vi "Autonomous.vi"() -> ()   [LabVIEW 2016]
doc: "This VI starts when autonomous period begins, and will automatically be terminated when it ends. You can carry out timed or sensor driven operations directly to I/O or to subsystems without needing to return to the caller."
uses:
  <vilib>/Rock Robotics/WPI/Solenoid/WPI_SolenoidValue.ctl
  <vilib>/Rock Robotics/Network Tables/NT Read String.vi
  <vilib>/Rock Robotics/Network Tables/NT Read Number.vi
  <vilib>/Rock Robotics/WPI/Solenoid/WPI_SolenoidSetEnum.vi
  Drive/Implementation/Drive Published Globals.vi
panel:
  in  "motor test time":dbl=1.0
  in  "Suckit":dbl=0.15 format="%#_13g"
  in  "Distance (ft) 2":dbl=3.0 format="%#_13g"
  in  "Distance (ft) 5":dbl=1.5
  in  "Distance (ft) 4":dbl=3.0
  in  "Distance (ft)":dbl=3.0 format="%#_13g"
  in  "Secs for flywheel spinup":dbl=0.3
  in  "Seconds to score":dbl=0.75
  in  "speed of backing up":dbl=0.3 format="%#_13g"
  in  "Seconds of backing up":dbl=2.0 format="%#_13g"
  in  "speed":dbl=-0.5 format="%#_13g"
  in  "Distance to go Forward":dbl=-11.658 format="%#_13g"
  in  "Score Goal Wait":dbl=0.5
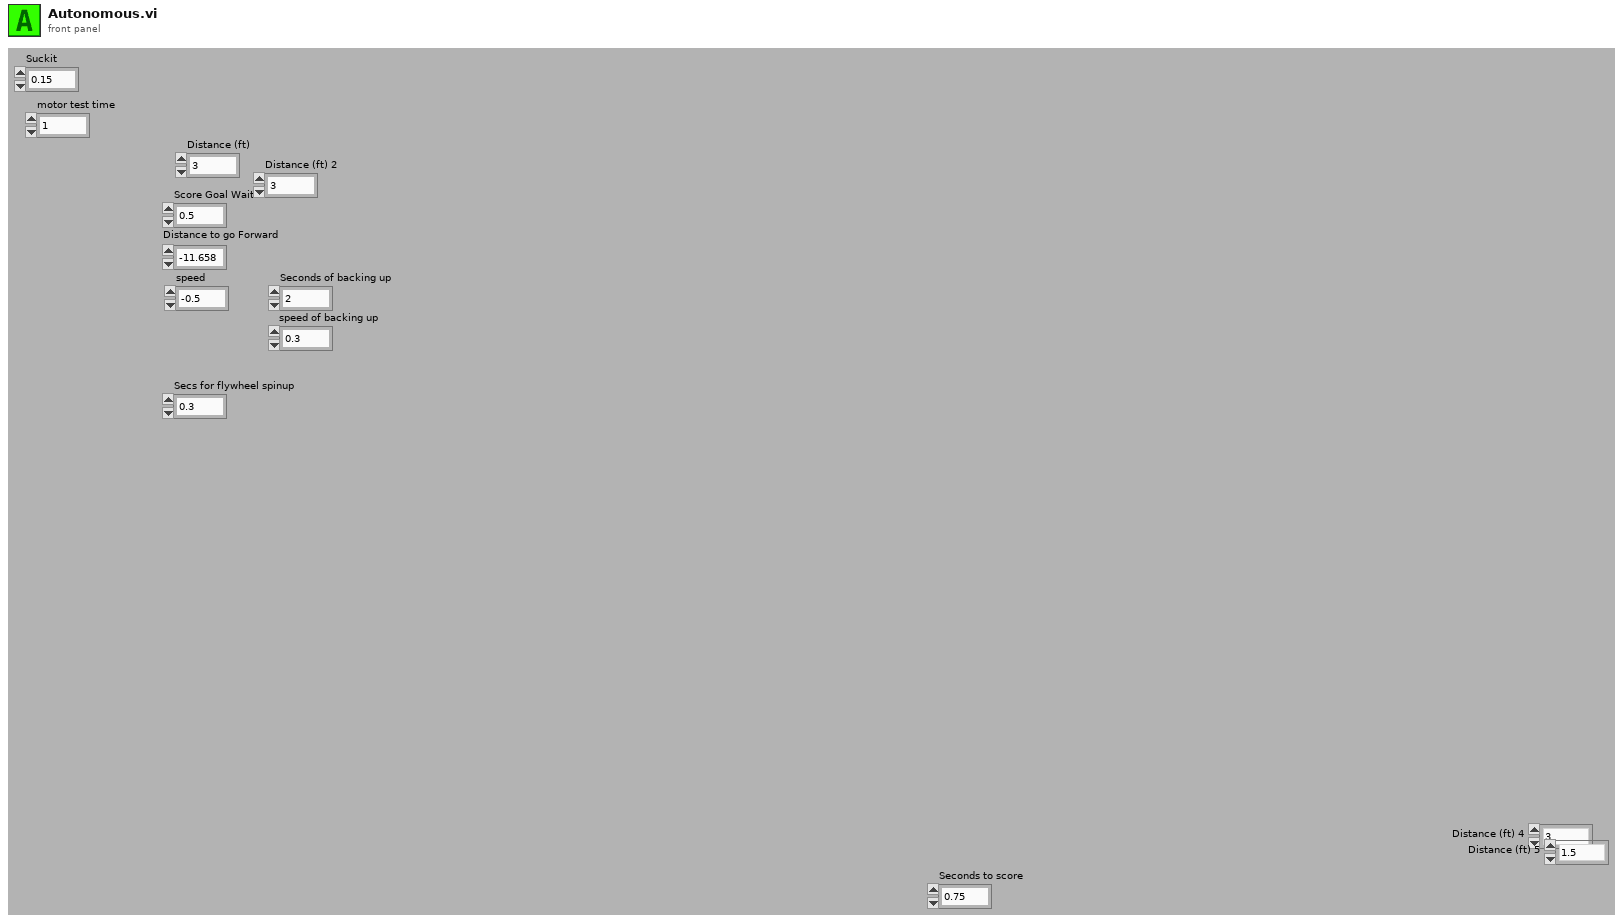
[diagram p1: front panel]
types:
  T1 = typedef "WPI_MotorControlDeviceRef.ctl" = cluster{"DeviceStatus":errorcluster, "Type":T2, "PWM":cluster{"PWM Channel":T3, "DeadBand":T4}, "CAN":cluster{"Device Number":u8, "SetOutput VI Ref":variant, "GetOutput VI Ref":variant, "Enable VI Ref":variant, "Disable VI Ref":variant, "Data":variant}, "Invert":bool}
  T2 = typedef "WPI_MotorControlType.ctl" = enum16{"PWM", "CAN"}
  T3 = typedef "FPGA_DIOPWMChannel.ctl" = enum8{"PWM 0", "PWM 1", "PWM 2", "PWM 3", "PWM 4", "PWM 5", "PWM 6", "PWM 7", "PWM 8", "PWM 9", "PWM MXP 0", "PWM MXP 1", "PWM MXP 2", "PWM MXP 3", "PWM MXP 4", "PWM MXP 5", "PWM MXP 6", "PWM MXP 7", "PWM MXP 8", "PWM MXP 9", "Invalid"}
  T4 = typedef "WPI_PWMDeadband.ctl" = cluster{"Name":string, "maxPositivePwm":i32, "minPositivePwm":i32, "centerPwm":i32, "maxNegativePwm":i32, "minNegativePwm":i32, "angularRange":u16}
  T5 = typedef "WPI_SolenoidDevRef.ctl" = cluster{"DevStatus":errorcluster, "Pneumatics Control Module":u8, "Forward Solenoid Channel":T6, "Reverse Solenoid Channel":T6}
  T6 = typedef "WPI_SolenoidChannel.ctl" = enum8{"Solenoid 0", "Solenoid 1", "Solenoid 2", "Solenoid 3", "Solenoid 4", "Solenoid 5", "Solenoid 6", "Solenoid 7", "Invalid"}
  T7 = typedef "WPI_SolenoidValue.ctl" = enum16{"Off", "On", "Forward", "Reverse"}
  T8 = typedef "Command Status Info.ctl" = cluster{"Name":string, "Status":T9, "notifier out":T10}
  T9 = typedef "Completion Status.ctl" = enum16{"Successful", "Aborted", "Incomplete"}
  T10 = typedef "Completion Notifier.ctl" = refnum<notifier>
  T11 = typedef "CTRE_PigeonIMU_DeviceRef.ctl" = cluster{"DeviceStatus":errorcluster, "Device Number":u8, "Type":T12, "Device ID":u32}
  T12 = typedef "CTRE_PigeonIMU_ConnectionType.ctl" = u32
  T13 = typedef "CTRE_PigeonIMU_GlobalStatus.ctl" = cluster{"PigeonState":T14, "FusedHeading":cluster{"Heading":dbl, "Valid?":bool, "Fusing?":bool}, "YPR":cluster{"Yaw":dbl, "Pitch":dbl, "Roll":dbl}, "Compass":cluster{"Heading":dbl, "Magnitude":dbl, "Absolute Heading":dbl}, "Accelerometer":cluster{"Biased":cluster{"X":i16, "Y":i16, "Z":i16, "Norm":i16}, "Angles":cluster{"XZ Tilt":dbl, "YZ Tilt":dbl, "XY Tilt":dbl}}, "Magnetometer":cluster{"Raw":cluster{"X":i16, "Y":i16, "Z":i16}, "Biased":cluster{"X":i16, "Y":i16, "Z":i16}}, "Gyro":cluster{"X":dbl, "Y":dbl, "Z":dbl, "Norm":dbl}, "6D Quaternian":cluster{"W":dbl, "X":dbl, "Y":dbl, "Z":dbl}, "Temp. (C)":dbl, "UpTime":u32, "StartupStatus":cluster{"ResetCount":i32, "ResetFlags":i32, "FirmwareVersion":i32, "HasReset?":bool}, "Calibration":cluster{"CurrentMode":T15, "LastCalError":i32, "CalBooting?":bool}, "CAN Error":errorcluster, "AccumGyro":cluster{"X":dbl, "Y":dbl, "Z":dbl}, "Usage Frame":u32}
  T14 = typedef "CTRE_PigeonIMU_PigeonState.ctl" = enum16{"NoComm", "Initializing", "Ready", "UserCalibration"}
  T15 = typedef "CTRE_PigeonIMU_CalibrationMode.ctl" = u16
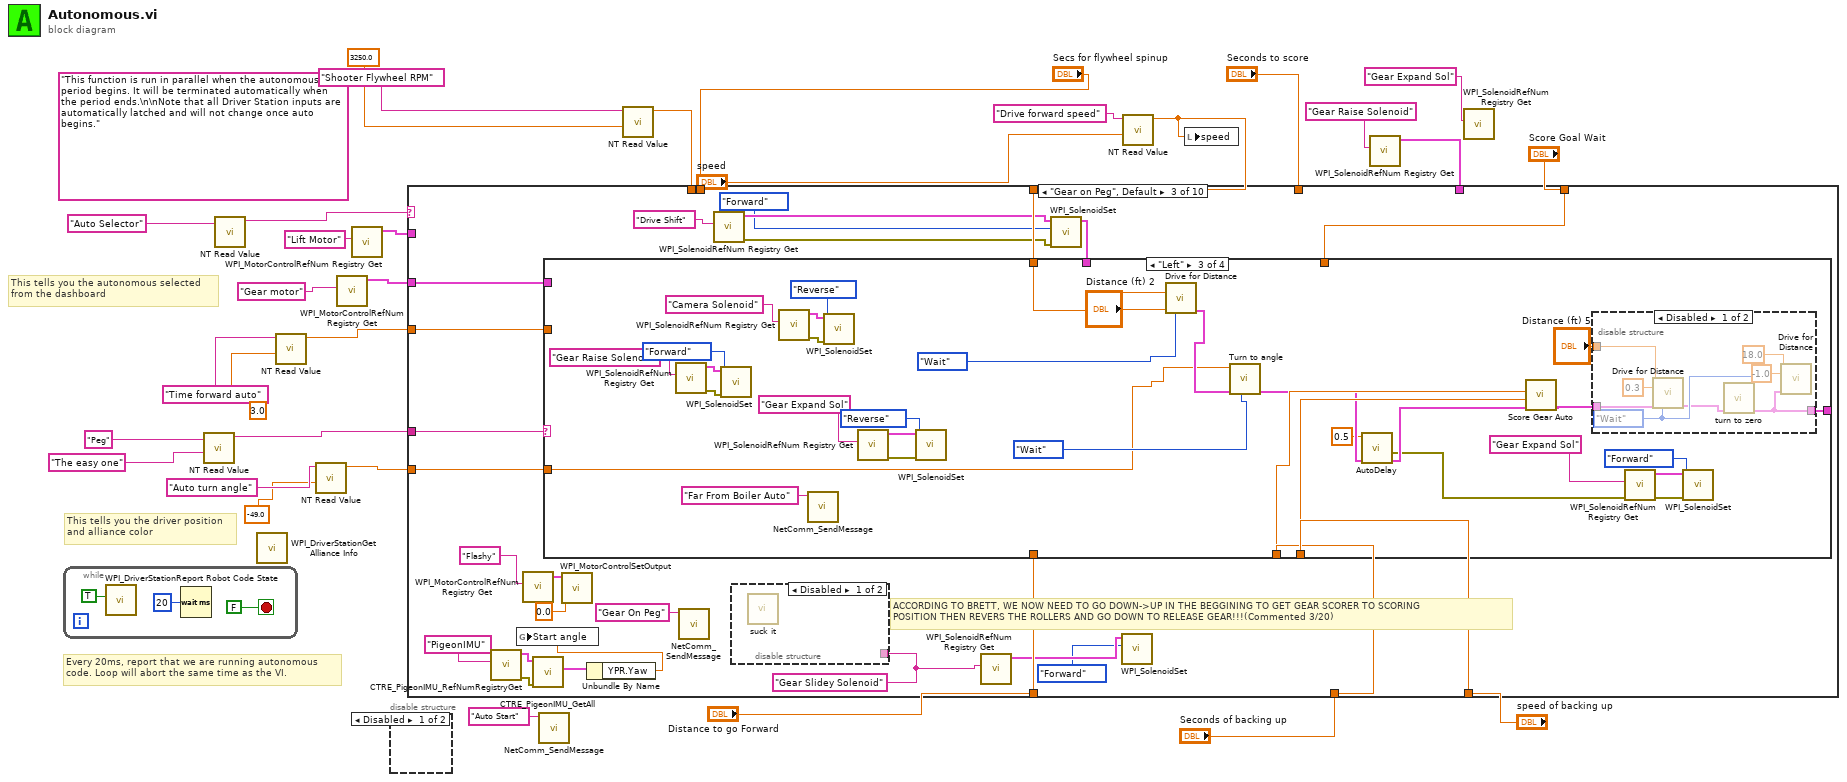
[diagram p0: block diagram]
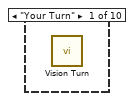
[diagram p3: hidden frame]
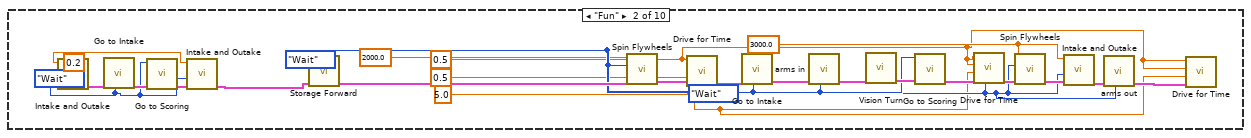
[diagram p4: hidden frame]
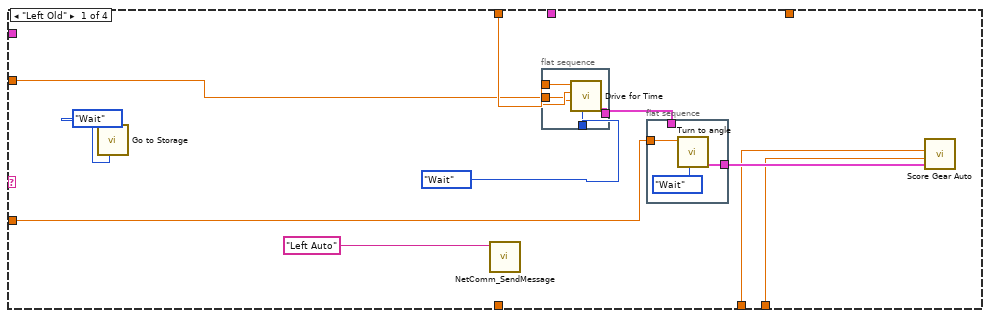
[diagram p6: hidden frame]
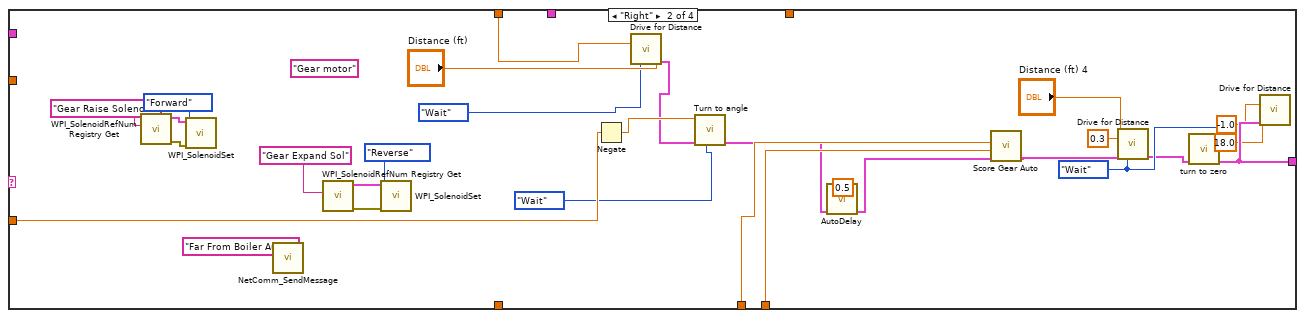
[diagram p7: hidden frame]
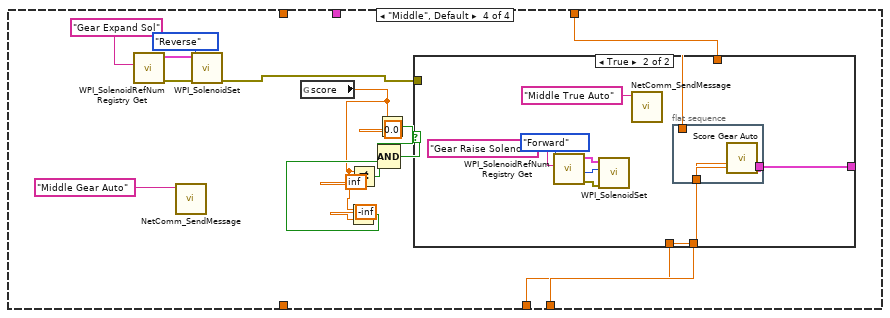
[diagram p9: hidden frame]
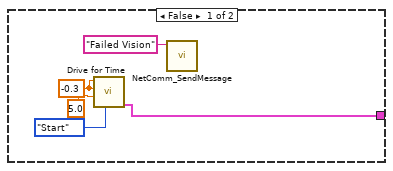
[diagram p10: hidden frame]
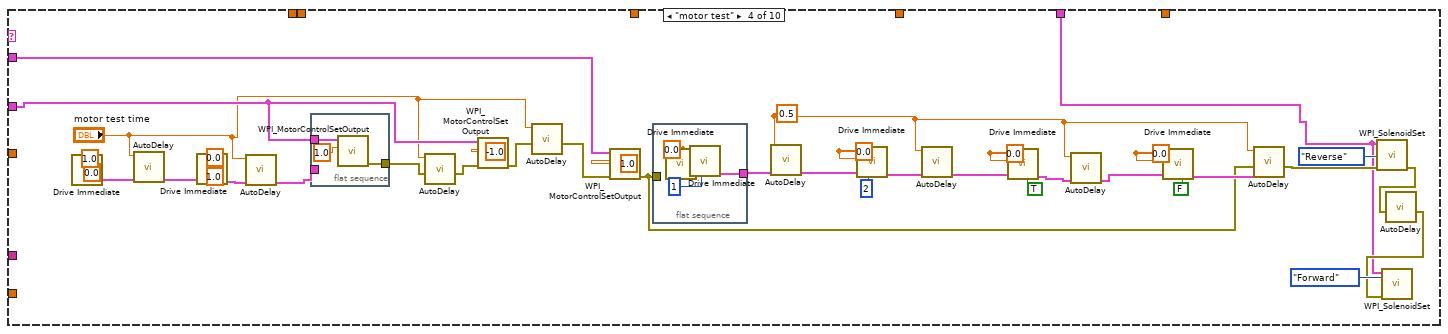
[diagram p11: hidden frame]
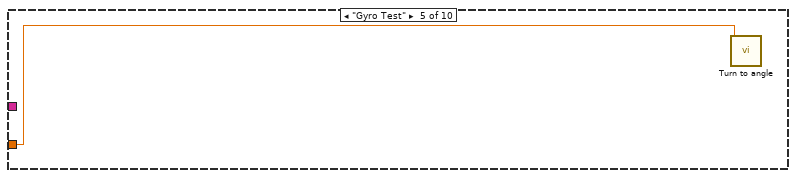
[diagram p12: hidden frame]
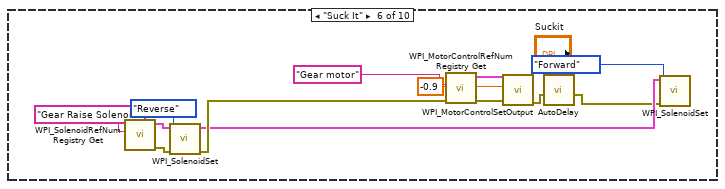
[diagram p13: hidden frame]
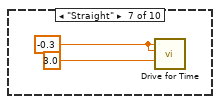
[diagram p14: hidden frame]
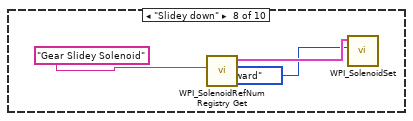
[diagram p15: hidden frame]
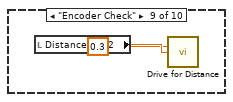
[diagram p16: hidden frame]
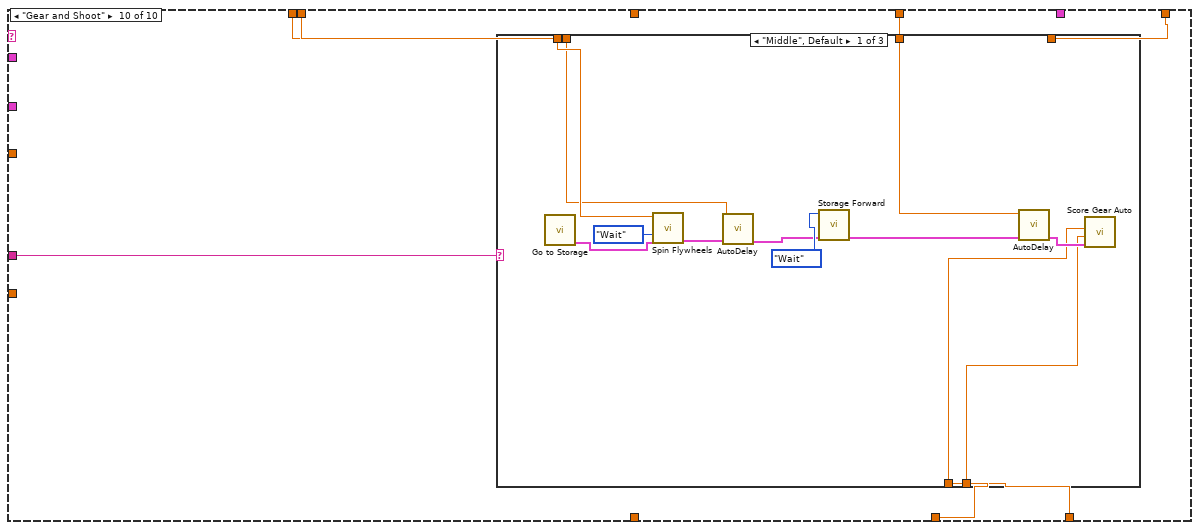
[diagram p17: hidden frame]
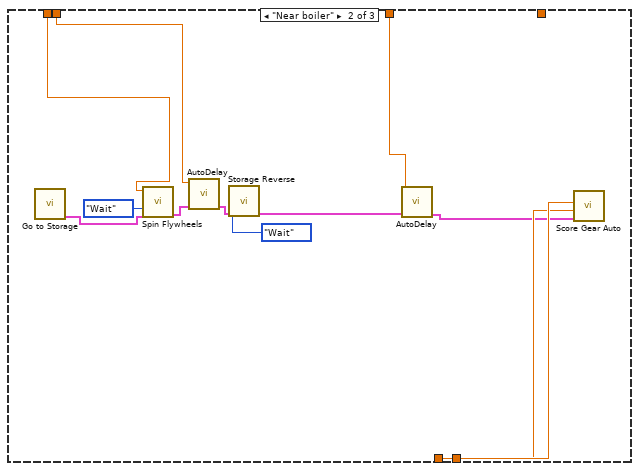
[diagram p18: hidden frame]
diagram:
  (unwired) "This function is run in parallel when the autonomous period begins. It will be terminated automatically when the period ends.\n\nNote that all Driver Station inputs are automatically latched and will not change once auto begins."
  # "This tells you the autonomous selected\nfrom the dashboard"
  # "Every 20ms, report that we are running autonomous\ncode. Loop will abort the same time as the VI."
  # "This tells you the driver position\nand alliance color"
  n1 = while {
    stop <- FALSE stop-if-true
    n2 = call <vilib>:"WPI_DriverStationReport Robot Code State.vi"("Autonomous"=TRUE) -> ()  [unwired: 10 in, 1 out]
    n3 = Wait (ms)(milliseconds to wait=u32 20) -> ()  [unwired: 1 out]
  }
  n4 = call-poly <vilib>:"NT Read Value.vi"("Default Value"="The easy one", "Name"="Peg") -> ("String"=w27:string)  [unwired: 8 in, 1 out]
  n5 = call-poly <vilib>:"NT Read Value.vi"("Name"="Auto Selector") -> ("String"=w30:string)  [unwired: 9 in, 1 out]
  n6 = call <vilib>:"WPI_DriverStationGet Alliance Info.vi"() -> ()  [unwired: 12 out]
  n7 = call-poly <vilib>:"NT Read Value.vi"("Default Value"=3.0, "Name"="Time forward auto") -> ("Numeric"=w15:dbl)  [unwired: 8 in, 1 out]
  n8 = call-poly <vilib>:"NT Read Value.vi"("Default Value"=-49.0, "Name"="Auto turn angle") -> ("Numeric"=w12:dbl)  [unwired: 8 in, 1 out]
  n9 = call <vilib>:"WPI_MotorControlRefNum Registry Get.vi"("refnum name"="Gear motor") -> ("MotorControlDevRef"=w7:T1)  [unwired: 9 in, 1 out]
  n10 = call <vilib>:"WPI_MotorControlRefNum Registry Get.vi"("refnum name"="Lift Motor") -> ("MotorControlDevRef"=w4:T1)  [unwired: 9 in, 1 out]
  n11 = disable-structure shown="Disabled" {
    frame Disabled {
    }
    frame Enabled {
    }
  }
  n12 = call <vilib>:"NetComm_SendMessage.vi"("Message"="Auto Start") -> ()  [unwired: 11 in]
  n13 = call-poly <vilib>:"NT Read Value.vi"("Default Value"=3250.0, "Name"="Shooter Flywheel RPM") -> ("Numeric"=w18:dbl)  [unwired: 8 in, 1 out]
  n14 = call-poly <vilib>:"NT Read Value.vi"("Default Value"="speed", "Name"="Drive forward speed") -> ("Numeric"=w9:dbl)  [unwired: 8 in, 1 out]
  n15 = local write "speed"(w9) -> ()
  n16 = call <vilib>:"WPI_SolenoidRefNum Registry Get.vi"("refnum name"="Gear Raise Solenoid") -> ("SolenoidDevRef"=w1:T5)  [unwired: 9 in, 1 out]
  n17 = case shown="\"Gear on Peg\", Default" w30 {
    tunnel: w27 -> [_ _ w84 _ _ _ _ _ _ w277]
    tunnel: w9 -> [_ _ w83 _ _ _ _ _ _ _]
    tunnel: "Distance to go Forward" -> [_ _ w82 _ _ _ _ _ _ _]
    tunnel: "speed of backing up" -> [_ _ w81 _ _ _ _ _ _ w275]
    tunnel: "Seconds of backing up" -> [_ _ w80 _ _ _ _ _ _ w276]
    tunnel: "Score Goal Wait" -> [_ _ w79 _ _ _ _ _ _ w274]
    tunnel: "Seconds to score" -> [_ _ _ _ _ _ _ _ _ w273]
    tunnel: "Secs for flywheel spinup" -> [_ _ _ _ _ _ _ _ _ w272]
    tunnel: w18 -> [_ _ _ _ _ _ _ _ _ w271]
    tunnel: w15 -> [_ _ w78 _ _ _ _ _ _ _]
    tunnel: w12 -> [_ _ w77 _ w249 _ _ _ _ _]
    tunnel: w7 -> [_ _ w71 w231 _ _ _ _ _ _]
    tunnel: w4 -> [_ _ _ w228 _ _ _ _ _ _]
    tunnel: w1 -> [_ _ _ w205 _ _ _ _ _ _]
    frame "Your Turn" {
      n18 = call "Vision Turn.vi"() -> ()  [unwired: 11 in, 1 out]
    }
    frame "Fun" {
      w36 = enum16{"Start", "Wait"}."Wait" ("Synchronication")
      w35 = 0.2 ("Speed")
      w47 = 3000.0 ("Speed RPM")
      w44 = enum16{"Start", "Wait"}."Wait" ("Synchronization")
      w41 = 5.0 ("Seconds")
      w42 = 0.5 ("Left Speed")
      w52 = enum16{"Start", "Wait"}."Wait" ("Synchronication")
      n19 = call "Intake and Outake.vi"("Synchronication"=w36, "Speed"=w35) -> ("Command Info Out"=w40:T8)  [unwired: 9 in]
      n20 = call "Go to Intake.vi"("Synchronication"=w36, "Command Info In"=w40) -> ("Command Info Out"=w38:T8)  [unwired: 9 in]
      n21 = call "Go to Scoring.vi"("Command Info In"=w38, "Synchronication"=w36) -> ("Command Info Out"=w37:T8)  [unwired: 9 in]
      n22 = call "Intake and Outake.vi"("Command Info In"=w37, "Synchronication"=w36, "Speed"=w35) -> ("Command Info Out"=w39:T8)  [unwired: 8 in]
      n23 = call "Storage Forward.vi"("Command Info In"=w39, "Synchronication"=w52) -> ("Command Info Out"=w58:T8)  [unwired: 9 in]
      n24 = call "Spin Flywheels.vi"("Command Info In"=w58, "Synchronication"=w52, "Speed RPM"=2000.0) -> ("Command Info Out"=w57:T8)  [unwired: 8 in]
      n25 = call "Drive for Time.vi"("Synchronization"=w52, "Command Info In"=w57, "Seconds"=w41, "Right Speed"=0.5, "Left Speed"=w42) -> ("Command Info Out"=w56:T8)  [unwired: 4 in, 2 out]
      n26 = call "Go to Intake.vi"("Synchronication"=w52, "Command Info In"=w56) -> ("Command Info Out"=w55:T8)  [unwired: 9 in]
      n27 = call "arms in.vi"("Synchronication"=w52, "Command Info In"=w55) -> ("Command Info Out"=w54:T8)  [unwired: 9 in]
      n28 = call "Vision Turn.vi"("Command Info In"=w54) -> ("Command Info Out"=w53:T8)  [unwired: 10 in]
      n29 = call "Go to Scoring.vi"("Command Info In"=w53, "Synchronication"=w52) -> ("Command Info Out"=w50:T8)  [unwired: 9 in]
      n30 = call "Drive for Time.vi"("Synchronization"=w44, "Command Info In"=w50, "Seconds"=w41, "Right Speed"=w42, "Left Speed"=w42) -> ("Command Info Out"=w48:T8)  [unwired: 4 in, 2 out]
      n31 = call "Spin Flywheels.vi"("Command Info In"=w48, "Synchronication"=w44, "Speed RPM"=w47) -> ("Command Info Out"=w46:T8)  [unwired: 8 in]
      n32 = call "Intake and Outake.vi"("Command Info In"=w46, "Synchronication"=w44, "Speed"=w47) -> ("Command Info Out"=w45:T8)  [unwired: 8 in]
      n33 = call "arms out.vi"("Synchronication"=w44, "Command Info In"=w45) -> ("Command Info Out"=w43:T8)  [unwired: 9 in]
      n34 = call "Drive for Time.vi"("Command Info In"=w43, "Seconds"=w41, "Right Speed"=w42, "Left Speed"=w42) -> ()  [unwired: 5 in, 3 out]
    }
    frame "Gear on Peg", Default {
      w62 = "Gear Slidey Solenoid" ("refnum name")
      # "ACCORDING TO BRETT, WE NOW NEED TO GO DOWN->UP IN THE BEGGINING TO GET GEAR SCORER TO SCORING \nPOSITION THEN REVERS THE ROLLERS AND GO DOWN TO RELEASE GEAR!!!(Commented 3/20)"
      n35 = call <vilib>:"CTRE_PigeonIMU_RefNumRegistryGet.vi"("refnum name"="PigeonIMU") -> ("error out"=w68:errorcluster, "PigeonIMUDevRef"=w67:T11)  [unwired: 9 in]
      n36 = call <vilib>:"WPI_MotorControlRefNum Registry Get.vi"("refnum name"="Flashy") -> ("MotorControlDevRef"=w60:T1)  [unwired: 9 in, 1 out]
      n37 = call <vilib>:"CTRE_PigeonIMU_GetAll.vi"("error in (no error)"=w68, "PigeonIMUDevRef"=w67) -> ("Get All"=w66:T13)  [unwired: 7 in, 2 out]
      n38 = call <vilib>:"WPI_MotorControlSetOutput.vi"("Output"=0.0, "MotorControlDevRef"=w60) -> ()  [unwired: 7 in, 3 out]
      n39 = Unbundle By Name(w66) -> ("YPR.Yaw"=w65:dbl)
      n40 = global write "Drive Published Globals.vi" "Start angle"(w65) -> ()
      n41 = call <vilib>:"NetComm_SendMessage.vi"("Message"="Gear On Peg") -> ()  [unwired: 11 in]
      n42 = call <vilib>:"WPI_SolenoidRefNum Registry Get.vi"("refnum name"="Drive Shift") -> ("error out"=w74:errorcluster, "SolenoidDevRef"=w75:T5)  [unwired: 9 in]
      n43 = disable-structure shown="Disabled" {
        disable-tunnel: w62 -> [_ _]
        frame Disabled {
          n44 = call "suck it.vi"() -> ()  [unwired: 12 in]
        }
        frame Enabled {
        }
      }
      n45 = call <vilib>:"WPI_SolenoidRefNum Registry Get.vi"("refnum name"=w62) -> ("SolenoidDevRef"=w64:T5)  [unwired: 9 in, 1 out]
      n46 = call-poly <vilib>:"WPI_SolenoidSet.vi"("error in (no error)"=w74, "Value"=WPI_SolenoidValue."Forward", "SolenoidDevRef"=w75) -> ("SolenoidDevRef"=w72:T5)  [unwired: 7 in, 1 out]
      n47 = case shown="\"Left\"" w84 {
        tunnel: w83 -> [w90 w113 w147 _]
        tunnel: w82 -> [_ _ _ _]
        tunnel: w81 -> [w93 w130 w162 w187]
        tunnel: w80 -> [w92 w129 w161 w186]
        tunnel: w79 -> [_ _ _ w185]
        tunnel: w78 -> [w89 _ _ _]
        tunnel: w77 -> [w91 w127 w140 _]
        tunnel: w72 -> [_ _ _ _]
        tunnel: w71 -> [_ _ _ _]
        tunnel: [_ w104 w141 _] -> _
        frame "Left Old" {
          n48 = call "Go to Storage.vi"("Synchronication"=enum16{"Start", "Wait"}."Wait") -> ()  [unwired: 10 in, 1 out]
          n49 = call <vilib>:"NetComm_SendMessage.vi"("Message"="Left Auto") -> ()  [unwired: 11 in]
          n50 = flat-sequence {
            tunnel: w90 -> [w101]
            tunnel: w89 -> [w100]
            tunnel: enum16{"Start", "Wait"}."Wait" ("Synchronication") -> [w99]
            tunnel: [w98] -> w87
            frame #0 {
              n51 = call "Drive for Time.vi"("Synchronization"=w99, "Seconds"=w100, "Right Speed"=w101, "Left Speed"=w101) -> ("Command Info Out"=w98:T8)  [unwired: 5 in, 2 out]
            }
          }
          n52 = flat-sequence {
            tunnel: [w97] -> w94
            tunnel: w91 -> [w95]
            tunnel: w87 -> [_]
            frame #0 {
              n53 = call "Turn to angle.vi"("Synchronication"=enum16{"Start", "Wait"}."Wait", "Angle"=w95) -> ("Command Info Out"=w97:T8)  [unwired: 9 in]
            }
          }
          n54 = call "Score Gear Auto.vi"("Command Info in"=w94, "speed of backing up"=w93, "Seconds of backing up"=w92) -> ()  [unwired: 8 in, 1 out]
        }
        frame "Right" {
          (unwired) "Gear motor" ("refnum name")
          w107 = enum16{"Start", "Wait"}."Wait" ("Synchronication")
          n55 = call <vilib>:"WPI_SolenoidRefNum Registry Get.vi"("refnum name"="Gear Raise Solenoid") -> ("error out"=w122:errorcluster, "SolenoidDevRef"=w123:T5)  [unwired: 9 in]
          n56 = call-poly <vilib>:"WPI_SolenoidSet.vi"("error in (no error)"=w122, "Value"=WPI_SolenoidValue."Forward", "SolenoidDevRef"=w123) -> ()  [unwired: 7 in, 2 out]
          n57 = call <vilib>:"NetComm_SendMessage.vi"("Message"="Far From Boiler Auto") -> ()  [unwired: 11 in]
          n58 = call <vilib>:"WPI_SolenoidRefNum Registry Get.vi"("refnum name"="Gear Expand Sol") -> ("error out"=w119:errorcluster, "SolenoidDevRef"=w118:T5)  [unwired: 9 in]
          n59 = call-poly <vilib>:"WPI_SolenoidSet.vi"("error in (no error)"=w119, "Value"=WPI_SolenoidValue."Reverse", "SolenoidDevRef"=w118) -> ()  [unwired: 7 in, 2 out]
          n60 = Negate(x=w127) -> (-x=w128:dbl)
          n61 = call "Drive for Distance.vi"("speed"=w113, "Distance (ft)"="Distance (ft)", "Synchronication"=enum16{"Start", "Wait"}."Wait") -> ("Command Info Out"=w111:T8)  [unwired: 12 in]
          n62 = call "Turn to angle.vi"("Synchronication"=enum16{"Start", "Wait"}."Wait", "Command Info In"=w111, "Angle"=w128) -> ("Command Info Out"=w116:T8)  [unwired: 8 in]
          n63 = call "AutoDelay.vi"("Command Info In"=w116, "Seconds to wait"=0.5) -> ("Command Info Out"=w115:T8)  [unwired: 8 in, 1 out]
          n64 = call "Score Gear Auto.vi"("Command Info in"=w115, "speed of backing up"=w130, "Seconds of backing up"=w129) -> ("Command Info Out"=w105:T8)  [unwired: 8 in]
          n65 = call "Drive for Distance.vi"("speed"=0.3, "Distance (ft)"="Distance (ft) 4", "Command Info In"=w105, "Synchronication"=w107) -> ("Command Info Out"=w106:T8)  [unwired: 11 in]
          n66 = call "turn to zero.vi"("Synchronication"=w107, "Command Info In"=w106) -> ("Command Info Out"=w104:T8)  [unwired: 9 in]
          n67 = call "Drive for Distance.vi"("speed"=-1.0, "Distance (ft)"=18.0, "Command Info In"=w104) -> ()  [unwired: 12 in, 1 out]
        }
        frame "Left" {
          n68 = call <vilib>:"WPI_SolenoidRefNum Registry Get.vi"("refnum name"="Gear Raise Solenoid") -> ("error out"=w156:errorcluster, "SolenoidDevRef"=w157:T5)  [unwired: 9 in]
          n69 = call-poly <vilib>:"WPI_SolenoidSet.vi"("error in (no error)"=w156, "Value"=WPI_SolenoidValue."Forward", "SolenoidDevRef"=w157) -> ()  [unwired: 7 in, 2 out]
          n70 = call <vilib>:"WPI_SolenoidRefNum Registry Get.vi"("refnum name"="Camera Solenoid") -> ("error out"=w138:errorcluster, "SolenoidDevRef"=w137:T5)  [unwired: 9 in]
          n71 = call <vilib>:"NetComm_SendMessage.vi"("Message"="Far From Boiler Auto") -> ()  [unwired: 11 in]
          n72 = call-poly <vilib>:"WPI_SolenoidSet.vi"("error in (no error)"=w138, "Value"=WPI_SolenoidValue."Reverse", "SolenoidDevRef"=w137) -> ()  [unwired: 7 in, 2 out]
          n73 = call <vilib>:"WPI_SolenoidRefNum Registry Get.vi"("refnum name"="Gear Expand Sol") -> ("error out"=w153:errorcluster, "SolenoidDevRef"=w152:T5)  [unwired: 9 in]
          n74 = call-poly <vilib>:"WPI_SolenoidSet.vi"("error in (no error)"=w153, "Value"=WPI_SolenoidValue."Reverse", "SolenoidDevRef"=w152) -> ()  [unwired: 7 in, 2 out]
          n75 = call "Drive for Distance.vi"("speed"=w147, "Distance (ft)"="Distance (ft) 2", "Synchronication"=enum16{"Start", "Wait"}."Wait") -> ("Command Info Out"=w145:T8)  [unwired: 12 in]
          n76 = call "Turn to angle.vi"("Synchronication"=enum16{"Start", "Wait"}."Wait", "Command Info In"=w145, "Angle"=w140) -> ("Command Info Out"=w150:T8)  [unwired: 8 in]
          n77 = call "AutoDelay.vi"("Command Info In"=w150, "Seconds to wait"=0.5) -> ("Command Info Out"=w149:T8, "error out (no error)"=w131:errorcluster)  [unwired: 8 in]
          n78 = call "Score Gear Auto.vi"("Command Info in"=w149, "speed of backing up"=w162, "Seconds of backing up"=w161) -> ("Command Info Out"=w142:T8)  [unwired: 8 in]
          n79 = disable-structure shown="Disabled" {
            disable-tunnel: "Distance (ft) 5" -> [w170 _]
            disable-tunnel: w142 -> [w166 _]
            disable-tunnel: [w165 _] -> w141
            frame Disabled {
              w168 = enum16{"Start", "Wait"}."Wait" ("Synchronication")
              n80 = call "Drive for Distance.vi"("speed"=0.3, "Distance (ft)"=w170, "Command Info In"=w166, "Synchronication"=w168) -> ("Command Info Out"=w167:T8)  [unwired: 11 in]
              n81 = call "turn to zero.vi"("Synchronication"=w168, "Command Info In"=w167) -> ("Command Info Out"=w165:T8)  [unwired: 9 in]
              n82 = call "Drive for Distance.vi"("speed"=-1.0, "Distance (ft)"=18.0, "Command Info In"=w165) -> ()  [unwired: 12 in, 1 out]
            }
            frame Enabled {
            }
          }
          n83 = call <vilib>:"WPI_SolenoidRefNum Registry Get.vi"("error in (no error)"=w131, "refnum name"="Gear Expand Sol") -> ("error out"=w133:errorcluster, "SolenoidDevRef"=w134:T5)  [unwired: 8 in]
          n84 = call-poly <vilib>:"WPI_SolenoidSet.vi"("error in (no error)"=w133, "Value"=WPI_SolenoidValue."Forward", "SolenoidDevRef"=w134) -> ()  [unwired: 7 in, 2 out]
        }
        frame "Middle", Default {
          n85 = call <vilib>:"WPI_SolenoidRefNum Registry Get.vi"("refnum name"="Gear Expand Sol") -> ("error out"=w174:errorcluster, "SolenoidDevRef"=w173:T5)  [unwired: 9 in]
          n86 = call <vilib>:"NetComm_SendMessage.vi"("Message"="Middle Gear Auto") -> ()  [unwired: 11 in]
          n87 = call-poly <vilib>:"WPI_SolenoidSet.vi"("error in (no error)"=w174, "Value"=WPI_SolenoidValue."Reverse", "SolenoidDevRef"=w173) -> ("error out"=w171:errorcluster)  [unwired: 7 in, 1 out]
          n88 = global read "Drive Published Globals.vi" "score"() -> (w178:dbl)
          n89 = Not Equal?(x=w178, y=-inf) -> (x != y?=w180:bool)
          n90 = Not Equal?(x=w178, y=inf) -> (x != y?=w179:bool)
          n91 = Not Equal?(x=w178, y=0.0) -> (x != y?=w182:bool)
          n92 = Compound Arithmetic op=AND(w182, w180, w179) -> (w183:bool)
          n93 = case shown="True" w183 {
            tunnel: w187 -> [_ w201]
            tunnel: w186 -> [_ w200]
            tunnel: w185 -> [_ w199]
            tunnel: [w189 w198] -> _
            tunnel: w171 -> [_ _]
            frame False {
              w192 = -0.3 ("Right Speed")
              n94 = call "Drive for Time.vi"("Synchronization"=enum16{"Start", "Wait"}."Start", "Seconds"=5.0, "Right Speed"=w192, "Left Speed"=w192) -> ("Command Info Out"=w189:T8)  [unwired: 5 in, 2 out]
              n95 = call <vilib>:"NetComm_SendMessage.vi"("Message"="Failed Vision") -> ()  [unwired: 11 in]
            }
            frame True {
              n96 = call <vilib>:"WPI_SolenoidRefNum Registry Get.vi"("refnum name"="Gear Raise Solenoid") -> ("error out"=w194:errorcluster, "SolenoidDevRef"=w195:T5)  [unwired: 9 in]
              n97 = call-poly <vilib>:"WPI_SolenoidSet.vi"("error in (no error)"=w194, "Value"=WPI_SolenoidValue."Forward", "SolenoidDevRef"=w195) -> ()  [unwired: 7 in, 2 out]
              n98 = call <vilib>:"NetComm_SendMessage.vi"("Message"="Middle True Auto") -> ()  [unwired: 11 in]
              n99 = flat-sequence {
                tunnel: w201 -> [w204]
                tunnel: w200 -> [w203]
                tunnel: w199 -> [_]
                tunnel: [w202] -> w198
                frame #0 {
                  n100 = call "Score Gear Auto.vi"("speed of backing up"=w204, "Seconds of backing up"=w203) -> ("Command Info Out"=w202:T8)  [unwired: 9 in]
                }
              }
            }
          }
        }
      }
      n101 = call-poly <vilib>:"WPI_SolenoidSet.vi"("Value"=WPI_SolenoidValue."Forward", "SolenoidDevRef"=w64) -> ()  [unwired: 8 in, 2 out]
    }
    frame "motor test" {
      w216 = 0.0 ("Left Setpoint")
      w220 = 0.0 ("Left Setpoint")
      w212 = 0.5 ("Seconds to wait")
      w224 = 0.0 ("Left Setpoint")
      n102 = call "Drive Immediate.vi"("Right Setpoint"=0.0, "Left Setpoint"=1.0) -> ("Command Info Out"=w241:T8)  [unwired: 9 in]
      n103 = call "AutoDelay.vi"("Command Info In"=w241, "Seconds to wait"="motor test time") -> ("Command Info Out"=w239:T8)  [unwired: 8 in, 1 out]
      n104 = call "Drive Immediate.vi"("Command Info In"=w239, "Right Setpoint"=1.0, "Left Setpoint"=0.0) -> ("Command Info Out"=w236:T8)  [unwired: 8 in]
      n105 = call "AutoDelay.vi"("Command Info In"=w236, "Seconds to wait"="motor test time") -> ("Command Info Out"=w235:T8)  [unwired: 8 in, 1 out]
      n106 = flat-sequence {
        tunnel: w231 -> [w248]
        tunnel: w235 -> [_]
        tunnel: [w247] -> w234
        frame #0 {
          n107 = call <vilib>:"WPI_MotorControlSetOutput.vi"("Output"=1.0, "MotorControlDevRef"=w248) -> ("error out"=w247:errorcluster)  [unwired: 7 in, 2 out]
        }
      }
      n108 = call "AutoDelay.vi"("error in (no error)"=w234, "Seconds to wait"="motor test time") -> ("error out (no error)"=w233:errorcluster)  [unwired: 8 in, 1 out]
      n109 = call <vilib>:"WPI_MotorControlSetOutput.vi"("error in (no error)"=w233, "Output"=-1.0, "MotorControlDevRef"=w231) -> ("error out"=w227:errorcluster)  [unwired: 6 in, 2 out]
      n110 = call "AutoDelay.vi"("error in (no error)"=w227, "Seconds to wait"="motor test time") -> ("error out (no error)"=w229:errorcluster)  [unwired: 8 in, 1 out]
      n111 = call <vilib>:"WPI_MotorControlSetOutput.vi"("error in (no error)"=w229, "Output"=1.0, "MotorControlDevRef"=w228) -> ("error out"=w210:errorcluster)  [unwired: 6 in, 2 out]
      n112 = flat-sequence {
        tunnel: w210 -> [_]
        tunnel: [w243] -> w223
        frame #0 {
          w245 = 0.0 ("Left Setpoint")
          n113 = call "Drive Immediate.vi"("Shift"=1, "Right Setpoint"=w245, "Left Setpoint"=w245) -> ("Command Info Out"=w243:T8)  [unwired: 8 in]
        }
      }
      n114 = call "Drive Immediate.vi"() -> ()  [unwired: 11 in, 1 out]
      n115 = call "AutoDelay.vi"("Command Info In"=w223, "Seconds to wait"=w212) -> ("Command Info Out"=w222:T8)  [unwired: 8 in, 1 out]
      n116 = call "Drive Immediate.vi"("Shift"=2, "Command Info In"=w222, "Right Setpoint"=w224, "Left Setpoint"=w224) -> ("Command Info Out"=w219:T8)  [unwired: 7 in]
      n117 = call "AutoDelay.vi"("Command Info In"=w219, "Seconds to wait"=w212) -> ("Command Info Out"=w221:T8)  [unwired: 8 in, 1 out]
      n118 = call "Drive Immediate.vi"("Brake"=TRUE, "Command Info In"=w221, "Right Setpoint"=w220, "Left Setpoint"=w220) -> ("Command Info Out"=w215:T8)  [unwired: 7 in]
      n119 = call "AutoDelay.vi"("Command Info In"=w215, "Seconds to wait"=w212) -> ("Command Info Out"=w214:T8)  [unwired: 8 in, 1 out]
      n120 = call "Drive Immediate.vi"("Brake"=FALSE, "Command Info In"=w214, "Right Setpoint"=w216, "Left Setpoint"=w216) -> ("Command Info Out"=w213:T8)  [unwired: 7 in]
      n121 = call "AutoDelay.vi"("Command Info In"=w213, "error in (no error)"=w210, "Seconds to wait"=w212) -> ("error out (no error)"=w211:errorcluster)  [unwired: 7 in, 1 out]
      n122 = call-poly <vilib>:"WPI_SolenoidSet.vi"("error in (no error)"=w211, "Value"=WPI_SolenoidValue."Reverse", "SolenoidDevRef"=w205) -> ("error out"=w207:errorcluster)  [unwired: 7 in, 1 out]
      n123 = call "AutoDelay.vi"("error in (no error)"=w207) -> ("error out (no error)"=w206:errorcluster)  [unwired: 9 in, 1 out]
      n124 = call-poly <vilib>:"WPI_SolenoidSet.vi"("error in (no error)"=w206, "Value"=WPI_SolenoidValue."Forward", "SolenoidDevRef"=w205) -> ()  [unwired: 7 in, 2 out]
    }
    frame "Gyro Test" {
      n125 = call "Turn to angle.vi"("Angle"=w249) -> ()  [unwired: 10 in, 1 out]
    }
    frame "Suck It" {
      n126 = call <vilib>:"WPI_SolenoidRefNum Registry Get.vi"("refnum name"="Gear Raise Solenoid") -> ("error out"=w255:errorcluster, "SolenoidDevRef"=w256:T5)  [unwired: 9 in]
      n127 = call-poly <vilib>:"WPI_SolenoidSet.vi"("error in (no error)"=w255, "Value"=WPI_SolenoidValue."Reverse", "SolenoidDevRef"=w256) -> ("error out"=w253:errorcluster, "SolenoidDevRef"=w251:T5)  [unwired: 7 in]
      n128 = call <vilib>:"WPI_MotorControlRefNum Registry Get.vi"("error in (no error)"=w253, "refnum name"="Gear motor") -> ("error out"=w262:errorcluster, "MotorControlDevRef"=w258:T1)  [unwired: 8 in]
      n129 = call <vilib>:"WPI_MotorControlSetOutput.vi"("error in (no error)"=w262, "Output"=-0.9, "MotorControlDevRef"=w258) -> ("error out"=w260:errorcluster)  [unwired: 6 in, 2 out]
      n130 = call "AutoDelay.vi"("error in (no error)"=w260, "Seconds to wait"="Suckit") -> ("error out (no error)"=w250:errorcluster)  [unwired: 8 in, 1 out]
      n131 = call-poly <vilib>:"WPI_SolenoidSet.vi"("error in (no error)"=w250, "Value"=WPI_SolenoidValue."Forward", "SolenoidDevRef"=w251) -> ()  [unwired: 7 in, 2 out]
    }
    frame "Straight" {
      w265 = -0.3 ("Left Speed")
      n132 = call "Drive for Time.vi"("Seconds"=3.0, "Right Speed"=w265, "Left Speed"=w265) -> ()  [unwired: 6 in, 3 out]
    }
    frame "Slidey down" {
      n133 = call <vilib>:"WPI_SolenoidRefNum Registry Get.vi"("refnum name"="Gear Slidey Solenoid") -> ("SolenoidDevRef"=w267:T5)  [unwired: 9 in, 1 out]
      n134 = call-poly <vilib>:"WPI_SolenoidSet.vi"("Value"=WPI_SolenoidValue."Forward", "SolenoidDevRef"=w267) -> ()  [unwired: 8 in, 2 out]
    }
    frame "Encoder Check" {
      n135 = local read "Distance (ft) 2"() -> (w270:dbl)
      n136 = call "Drive for Distance.vi"("speed"=0.3, "Distance (ft)"=w270) -> ()  [unwired: 13 in, 1 out]
    }
    frame "Gear and Shoot" {
      n137 = case shown="\"Middle\", Default" w277 {
        tunnel: w276 -> [w283 w300 _]
        tunnel: w275 -> [w284 w299 _]
        tunnel: w274 -> [_ _ _]
        tunnel: w273 -> [w278 w296 _]
        tunnel: w272 -> [w285 w292 _]
        tunnel: w271 -> [w286 w295 _]
        frame "Middle", Default {
          n138 = call "Go to Storage.vi"() -> ("Command Info Out"=w288:T8)  [unwired: 11 in]
          n139 = call "Spin Flywheels.vi"("Command Info In"=w288, "Synchronication"=enum16{"Start", "Wait"}."Wait", "Speed RPM"=w286) -> ("Command Info Out"=w282:T8)  [unwired: 8 in]
          n140 = call "AutoDelay.vi"("Command Info In"=w282, "Seconds to wait"=w285) -> ("Command Info Out"=w280:T8)  [unwired: 8 in, 1 out]
          n141 = call "Storage Forward.vi"("Command Info In"=w280, "Synchronication"=enum16{"Start", "Wait"}."Wait") -> ("Command Info Out"=w279:T8)  [unwired: 9 in]
          n142 = call "AutoDelay.vi"("Command Info In"=w279, "Seconds to wait"=w278) -> ("Command Info Out"=w287:T8)  [unwired: 8 in, 1 out]
          n143 = call "Score Gear Auto.vi"("Command Info in"=w287, "speed of backing up"=w284, "Seconds of backing up"=w283) -> ()  [unwired: 8 in, 1 out]
        }
        frame "Near boiler" {
          n144 = call "Go to Storage.vi"() -> ("Command Info Out"=w298:T8)  [unwired: 11 in]
          n145 = call "Spin Flywheels.vi"("Command Info In"=w298, "Synchronication"=enum16{"Start", "Wait"}."Wait", "Speed RPM"=w295) -> ("Command Info Out"=w294:T8)  [unwired: 8 in]
          n146 = call "AutoDelay.vi"("Command Info In"=w294, "Seconds to wait"=w292) -> ("Command Info Out"=w293:T8)  [unwired: 8 in, 1 out]
          n147 = call "Storage Reverse.vi"("Command Info In"=w293, "Synchronication"=enum16{"Start", "Wait"}."Wait") -> ("Command Info Out"=w291:T8)  [unwired: 9 in]
          n148 = call "AutoDelay.vi"("Command Info In"=w291, "Seconds to wait"=w296) -> ("Command Info Out"=w290:T8)  [unwired: 8 in, 1 out]
          n149 = call "Score Gear Auto.vi"("Command Info in"=w290, "speed of backing up"=w299, "Seconds of backing up"=w300) -> ()  [unwired: 8 in, 1 out]
        }
        frame "Not an option" {
        }
      }
    }
  }
  n150 = call <vilib>:"WPI_SolenoidRefNum Registry Get.vi"("refnum name"="Gear Expand Sol") -> ()  [unwired: 9 in, 2 out]
